vi "Backpressure - level-aware.vi"(8 "error in (no error)":errorcluster) -> (0 "error out":errorcluster)   [LabVIEW 2026, in "Tests.lvlib"]
doc: "Unit test (Caraya): verifies ApplyBackPressure's LevelAware policy, including the fast-path and scan oracle.\nOn a full bounded queue, asserts the victim is the oldest least-severe non-protected Statement (protected = level at or more severe than ERROR; floor = TRACE), that the incoming loses severity ties (strict worstSev > incoming), and that worstSeverityOut is recomputed over the survivors on the scan branch and passed through on the fast path.\nTests.lvlib, friend of Lumberjack.lvlib; unit tier.\n\nImplements LMBR-T-049 -> SRS-057. Assert-level IDs: Test-ID-Assert-Checklist.md."
uses:
  Tests.lvlib
  src/TypeDefs/Statement.ctl
  src/TypeDefs/Severity.ctl
  src/TypeDefs/DropPolicy.ctl
  <vilib>/addons/_JKI Toolkits/Caraya/classes/Assert/Assert Equal Value_Variant.vi
  <vilib>/addons/_JKI Toolkits/Caraya/classes/Test/Test.lvclass
  src/Lumberjack.lvlib
  <vilib>/addons/_JKI Toolkits/Caraya/classes/Assert/Assert.lvclass
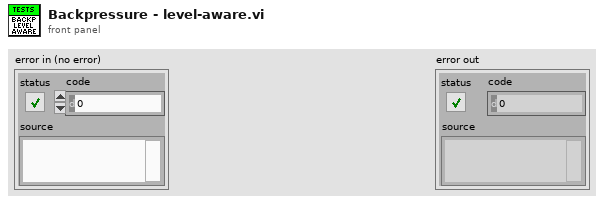
[diagram p1: front panel]
types:
  T1 = typedef "Lumberjack.lvlib/Statement.ctl" = cluster{"timestamp":timestamp, "level":T2, "sourceTag":string, "originVI":string, "message":string}
  T2 = typedef "Lumberjack.lvlib/Severity.ctl" = enum16{"OFF", "FATAL", "ERROR", "WARN", "INFO", "DEBUG", "TRACE", "ALL"}
  T3 = typedef "Lumberjack.lvlib/DropPolicy.ctl" = enum16{"DropOldest", "DropNewest", "LevelAware"}
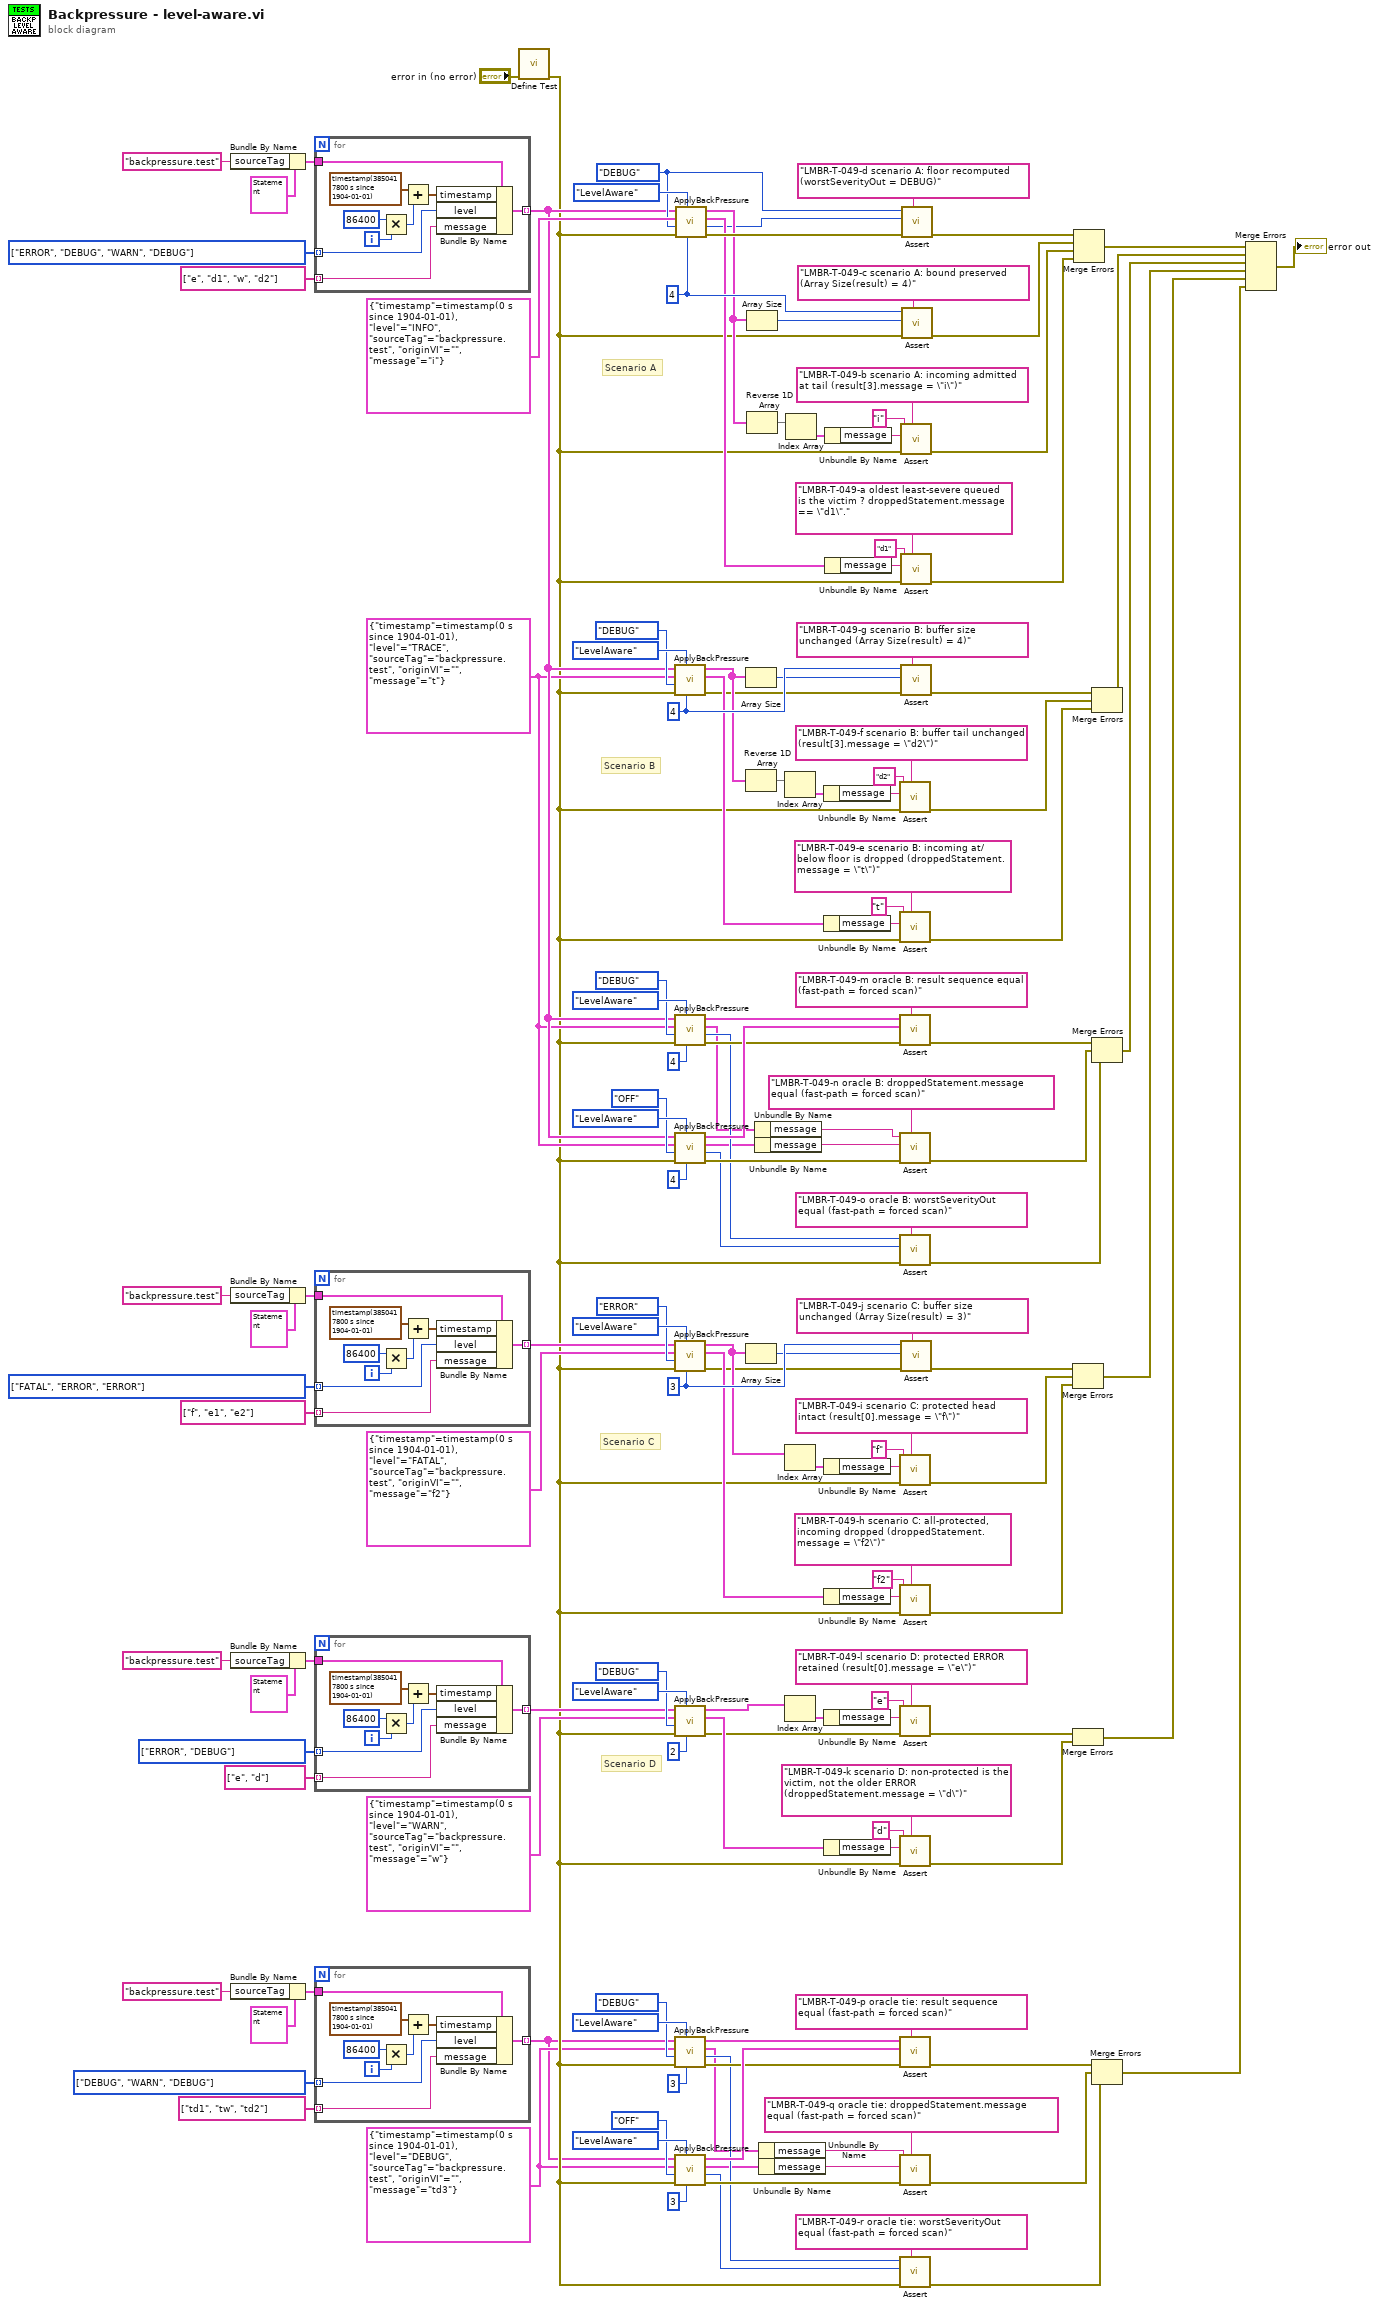
[diagram p0: block diagram]
diagram:
  w2 = T1 {"timestamp"=timestamp(0 s since 1904-01-01), "level"=enum."DEBUG", "sourceTag"="backpressure.test", "originVI"="", "message"="td3"} ("incoming")
  w12 = T2[] [enum."DEBUG", enum."WARN", enum."DEBUG"] items=["OFF", "FATAL", "ERROR", "WARN", "INFO", "DEBUG", "TRACE", "ALL"]
  w76 = T2[] [enum."ERROR", enum."DEBUG"] items=["OFF", "FATAL", "ERROR", "WARN", "INFO", "DEBUG", "TRACE", "ALL"]
  w98 = 3 ("queueBound")
  w101 = T2[] [enum."FATAL", enum."ERROR", enum."ERROR"] items=["OFF", "FATAL", "ERROR", "WARN", "INFO", "DEBUG", "TRACE", "ALL"]
  w51 = T1 {"timestamp"=timestamp(0 s since 1904-01-01), "level"=enum."TRACE", "sourceTag"="backpressure.test", "originVI"="", "message"="t"} ("incoming")
  w125 = 4 ("queueBound")
  w130 = T2[] [enum."ERROR", enum."DEBUG", enum."WARN", enum."DEBUG"] items=["OFF", "FATAL", "ERROR", "WARN", "INFO", "DEBUG", "TRACE", "ALL"]
  w129 = Severity."DEBUG" ("worstSeverityIn")
  w148 = 4 ("queueBound")
  # "Scenario D"
  # "Scenario C"
  # "Scenario B"
  # "Scenario A"
  n1 = Bundle By Name(cluster=T1 {"timestamp"=timestamp(0 s since 1904-01-01), "level"=enum."INFO", "sourceTag"="", "originVI"="", "message"=""} ("Statement"), "sourceTag"="backpressure.test") -> (w153:T1)
  n2 = Bundle By Name(cluster=T1 {"timestamp"=timestamp(0 s since 1904-01-01), "level"=enum."INFO", "sourceTag"="", "originVI"="", "message"=""} ("Statement"), "sourceTag"="backpressure.test") -> (w103:T1)
  n3 = Bundle By Name(cluster=T1 {"timestamp"=timestamp(0 s since 1904-01-01), "level"=enum."INFO", "sourceTag"="", "originVI"="", "message"=""} ("Statement"), "sourceTag"="backpressure.test") -> (w78:T1)
  n4 = Bundle By Name(cluster=T1 {"timestamp"=timestamp(0 s since 1904-01-01), "level"=enum."INFO", "sourceTag"="", "originVI"="", "message"=""} ("Statement"), "sourceTag"="backpressure.test") -> (w14:T1)
  n5 = for {
    tunnel: w153 -> [w162]
    tunnel: string[] ["e", "d1", "w", "d2"] -> [w159] mode=indexing
    tunnel: [w158] -> w52 mode=indexing
    tunnel: w130 -> [w157] mode=indexing
    i -> [w160]
    n6 = Multiply(x=86400, y=w160) -> (x*y=w164:i32)
    n7 = Add(x=timestamp(3850417800 s since 1904-01-01), y=w164) -> (x+y=w161:timestamp)
    n8 = Bundle By Name(cluster=w162, "timestamp"=w161, "level"=w157, "message"=w159) -> (w158:T1)
  }
  n9 = for {
    tunnel: w103 -> [w171]
    tunnel: string[] ["f", "e1", "e2"] -> [w168] mode=indexing
    tunnel: [w167] -> w84 mode=indexing
    tunnel: w101 -> [w166] mode=indexing
    i -> [w169]
    n10 = Multiply(x=86400, y=w169) -> (x*y=w173:i32)
    n11 = Add(x=timestamp(3850417800 s since 1904-01-01), y=w173) -> (x+y=w170:timestamp)
    n12 = Bundle By Name(cluster=w171, "timestamp"=w170, "level"=w166, "message"=w168) -> (w167:T1)
  }
  n13 = for {
    tunnel: w78 -> [w180]
    tunnel: string[] ["e", "d"] -> [w177] mode=indexing
    tunnel: [w176] -> w62 mode=indexing
    tunnel: w76 -> [w175] mode=indexing
    i -> [w178]
    n14 = Multiply(x=86400, y=w178) -> (x*y=w182:i32)
    n15 = Add(x=timestamp(3850417800 s since 1904-01-01), y=w182) -> (x+y=w179:timestamp)
    n16 = Bundle By Name(cluster=w180, "timestamp"=w179, "level"=w175, "message"=w177) -> (w176:T1)
  }
  n17 = for {
    tunnel: w14 -> [w189]
    tunnel: string[] ["td1", "tw", "td2"] -> [w186] mode=indexing
    tunnel: [w185] -> w1 mode=indexing
    tunnel: w12 -> [w184] mode=indexing
    i -> [w187]
    n18 = Multiply(x=86400, y=w187) -> (x*y=w191:i32)
    n19 = Add(x=timestamp(3850417800 s since 1904-01-01), y=w191) -> (x+y=w188:timestamp)
    n20 = Bundle By Name(cluster=w189, "timestamp"=w188, "level"=w184, "message"=w186) -> (w185:T1)
  }
  n21 = call <vilib>:"Define Test.vi"("error in (no error)"="error in (no error)") -> ("error out"=w11:errorcluster)  [unwired: 9 in, 1 out]
  n22 = call "ApplyBackPressure.vi"("queueBound"=w125, "DropPolicy"=DropPolicy."LevelAware", "error in (no error)"=w11, "worstSeverityIn"=Severity."DEBUG", "incoming"=w51, "pending"=w52) -> ("error out"=w106:errorcluster, "droppedStatement"=w121:T1, "result"=w114:T1[])  [unwired: 1 in, 2 out]
  n23 = call "ApplyBackPressure.vi"("queueBound"=4, "DropPolicy"=DropPolicy."LevelAware", "error in (no error)"=w11, "worstSeverityIn"=Severity."DEBUG", "incoming"=w51, "pending"=w52) -> ("error out"=w47:errorcluster, "worstSeverityOut"=w43:T2, "droppedStatement"=w10:T1, "result"=w49:T1[])  [unwired: 1 in, 1 out]
  n24 = call "ApplyBackPressure.vi"("queueBound"=4, "DropPolicy"=DropPolicy."LevelAware", "error in (no error)"=w11, "worstSeverityIn"=Severity."OFF", "incoming"=w51, "pending"=w52) -> ("error out"=w45:errorcluster, "worstSeverityOut"=w42:T2, "droppedStatement"=w9:T1, "result"=w48:T1[])  [unwired: 1 in, 1 out]
  n25 = call "ApplyBackPressure.vi"("queueBound"=w98, "DropPolicy"=DropPolicy."LevelAware", "error in (no error)"=w11, "worstSeverityIn"=Severity."ERROR", "incoming"=T1 {"timestamp"=timestamp(0 s since 1904-01-01), "level"=enum."FATAL", "sourceTag"="backpressure.test", "originVI"="", "message"="f2"}, "pending"=w84) -> ("error out"=w81:errorcluster, "droppedStatement"=w94:T1, "result"=w82:T1[])  [unwired: 1 in, 2 out]
  n26 = call "ApplyBackPressure.vi"("queueBound"=2, "DropPolicy"=DropPolicy."LevelAware", "error in (no error)"=w11, "worstSeverityIn"=Severity."DEBUG", "incoming"=T1 {"timestamp"=timestamp(0 s since 1904-01-01), "level"=enum."WARN", "sourceTag"="backpressure.test", "originVI"="", "message"="w"}, "pending"=w62) -> ("error out"=w59:errorcluster, "droppedStatement"=w71:T1, "result"=w60:T1[])  [unwired: 1 in, 2 out]
  n27 = call "ApplyBackPressure.vi"("queueBound"=3, "DropPolicy"=DropPolicy."LevelAware", "error in (no error)"=w11, "worstSeverityIn"=Severity."DEBUG", "incoming"=w2, "pending"=w1) -> ("error out"=w27:errorcluster, "worstSeverityOut"=w23:T2, "droppedStatement"=w4:T1, "result"=w29:T1[])  [unwired: 1 in, 1 out]
  n28 = call "ApplyBackPressure.vi"("queueBound"=3, "DropPolicy"=DropPolicy."LevelAware", "error in (no error)"=w11, "worstSeverityIn"=Severity."OFF", "incoming"=w2, "pending"=w1) -> ("error out"=w25:errorcluster, "worstSeverityOut"=w22:T2, "droppedStatement"=w6:T1, "result"=w28:T1[])  [unwired: 1 in, 1 out]
  n29 = call "ApplyBackPressure.vi"("queueBound"=w148, "DropPolicy"=DropPolicy."LevelAware", "error in (no error)"=w11, "worstSeverityIn"=w129, "incoming"=T1 {"timestamp"=timestamp(0 s since 1904-01-01), "level"=enum."INFO", "sourceTag"="backpressure.test", "originVI"="", "message"="i"}, "pending"=w52) -> ("error out"=w150:errorcluster, "worstSeverityOut"=w128:T2, "droppedStatement"=w143:T1, "result"=w134:T1[])  [unwired: 1 in, 1 out]
  n30 = Array Size(array=w114) -> (size(s)=w124:i32)
  n31 = Reverse 1D Array(array=w114) -> (reversed array=w119:T1[])
  n32 = Array Size(array=w82) -> (size(s)=w97:i32)
  n33 = Array Size(array=w134) -> (size(s)=w147:i32)
  n34 = Reverse 1D Array(array=w134) -> (reversed array=w139:T1[])
  n35 = Unbundle By Name(w10) -> ("message"=w7:string)
  n36 = Unbundle By Name(w9) -> ("message"=w8:string)
  n37 = Unbundle By Name(w4) -> ("message"=w3:string)
  n38 = Unbundle By Name(w6) -> ("message"=w5:string)
  n39 = Index Array(array=w119) -> (element=w115:T1)  [unwired: 1 in]
  n40 = Index Array(array=w82) -> (element=w88:T1)  [unwired: 1 in]
  n41 = Index Array(array=w60) -> (element=w66:T1)  [unwired: 1 in]
  n42 = Index Array(array=w139) -> (element=w135:T1)  [unwired: 1 in]
  n43 = Unbundle By Name(w115) -> ("message"=w116:string)
  n44 = Unbundle By Name(w121) -> ("message"=w120:string)
  n45 = Unbundle By Name(w88) -> ("message"=w89:string)
  n46 = Unbundle By Name(w94) -> ("message"=w93:string)
  n47 = Unbundle By Name(w66) -> ("message"=w67:string)
  n48 = Unbundle By Name(w71) -> ("message"=w70:string)
  n49 = Unbundle By Name(w135) -> ("message"=w136:string)
  n50 = Unbundle By Name(w143) -> ("message"=w142:string)
  n51 = call-poly <vilib>:"Assert.vi"("Label"="LMBR-T-049-f scenario B: buffer tail unchanged (result[3].message = \"d2\")" ("sourceTag"), "error in (no error)"=w11, "Actual"=w116, "Expected"="d2") -> ("error out"=w111:errorcluster)  [unwired: 6 in, 1 out]
  n52 = call-poly <vilib>:"Assert.vi"("Label"="LMBR-T-049-e scenario B: incoming at/below floor is dropped (droppedStatement.message = \"t\")" ("sourceTag"), "error in (no error)"=w11, "Actual"=w120, "Expected"="t") -> ("error out"=w110:errorcluster)  [unwired: 6 in, 1 out]
  n53 = call-poly <vilib>:"Assert.vi"("Label"="LMBR-T-049-m oracle B: result sequence equal (fast-path = forced scan)" ("sourceTag"), "error in (no error)"=w47, "Actual"=w48, "Expected"=w49) -> ("error out"=w41:errorcluster)  [unwired: 6 in, 1 out]
  n54 = call-poly <vilib>:"Assert.vi"("Label"="LMBR-T-049-n oracle B: droppedStatement.message equal (fast-path = forced scan)" ("sourceTag"), "error in (no error)"=w45, "Actual"=w8, "Expected"=w7) -> ("error out"=w40:errorcluster)  [unwired: 6 in, 1 out]
  n55 = call-poly <vilib>:"Assert.vi"("Label"="LMBR-T-049-o oracle B: worstSeverityOut equal (fast-path = forced scan)" ("sourceTag"), "error in (no error)"=w11, "Actual"=w42, "Expected"=w43) -> ("error out"=w39:errorcluster)  [unwired: 6 in, 1 out]
  n56 = call-poly <vilib>:"Assert.vi"("Label"="LMBR-T-049-i scenario C: protected head intact (result[0].message = \"f\")" ("sourceTag"), "error in (no error)"=w11, "Actual"=w89, "Expected"="f") -> ("error out"=w87:errorcluster)  [unwired: 6 in, 1 out]
  n57 = call-poly <vilib>:"Assert.vi"("Label"="LMBR-T-049-h scenario C: all-protected, incoming dropped (droppedStatement.message = \"f2\")" ("sourceTag"), "error in (no error)"=w11, "Actual"=w93, "Expected"="f2") -> ("error out"=w86:errorcluster)  [unwired: 6 in, 1 out]
  n58 = call-poly <vilib>:"Assert.vi"("Label"="LMBR-T-049-l scenario D: protected ERROR retained (result[0].message = \"e\")" ("sourceTag"), "error in (no error)"=w59, "Actual"=w67, "Expected"="e") -> ("error out"=w65:errorcluster)  [unwired: 6 in, 1 out]
  n59 = call-poly <vilib>:"Assert.vi"("Label"="LMBR-T-049-k scenario D: non-protected is the victim, not the older ERROR (droppedStatement.message = \"d\")" ("sourceTag"), "error in (no error)"=w11, "Actual"=w70, "Expected"="d") -> ("error out"=w64:errorcluster)  [unwired: 6 in, 1 out]
  n60 = call-poly <vilib>:"Assert.vi"("Label"="LMBR-T-049-p oracle tie: result sequence equal (fast-path = forced scan)" ("sourceTag"), "error in (no error)"=w27, "Actual"=w28, "Expected"=w29) -> ("error out"=w21:errorcluster)  [unwired: 6 in, 1 out]
  n61 = call-poly <vilib>:"Assert.vi"("Label"="LMBR-T-049-q oracle tie: droppedStatement.message equal (fast-path = forced scan)" ("sourceTag"), "error in (no error)"=w25, "Actual"=w5, "Expected"=w3) -> ("error out"=w20:errorcluster)  [unwired: 6 in, 1 out]
  n62 = call-poly <vilib>:"Assert.vi"("Label"="LMBR-T-049-r oracle tie: worstSeverityOut equal (fast-path = forced scan)" ("sourceTag"), "error in (no error)"=w11, "Actual"=w22, "Expected"=w23) -> ("error out"=w19:errorcluster)  [unwired: 6 in, 1 out]
  n63 = call-poly <vilib>:"Assert.vi"("Label"="LMBR-T-049-b scenario A: incoming admitted at tail (result[3].message = \"i\")" ("sourceTag"), "error in (no error)"=w11, "Actual"=w136, "Expected"="i") -> ("error out"=w133:errorcluster)  [unwired: 6 in, 1 out]
  n64 = call-poly <vilib>:"Assert.vi"("Label"="LMBR-T-049-a oldest least-severe queued is the victim ? droppedStatement.message == \"d1\"." ("sourceTag"), "error in (no error)"=w11, "Actual"=w142, "Expected"="d1") -> ("error out"=w132:errorcluster)  [unwired: 6 in, 1 out]
  n65 = call-poly <vilib>:"Assert.vi"("Label"="LMBR-T-049-g scenario B: buffer size unchanged (Array Size(result) = 4)" ("sourceTag"), "error in (no error)"=w106, "Actual"=w124, "Expected"=w125) -> ("error out"=w112:errorcluster)  [unwired: 6 in, 1 out]
  n66 = call-poly <vilib>:"Assert.vi"("Label"="LMBR-T-049-j scenario C: buffer size unchanged (Array Size(result) = 3)" ("sourceTag"), "error in (no error)"=w81, "Actual"=w97, "Expected"=w98) -> ("error out"=w92:errorcluster)  [unwired: 6 in, 1 out]
  n67 = call-poly <vilib>:"Assert.vi"("Label"="LMBR-T-049-d scenario A: floor recomputed (worstSeverityOut = DEBUG)" ("sourceTag"), "error in (no error)"=w150, "Actual"=w128, "Expected"=w129) -> ("error out"=w141:errorcluster)  [unwired: 6 in, 1 out]
  n68 = call-poly <vilib>:"Assert.vi"("Label"="LMBR-T-049-c scenario A: bound preserved (Array Size(result) = 4)" ("sourceTag"), "error in (no error)"=w11, "Actual"=w147, "Expected"=w148) -> ("error out"=w140:errorcluster)  [unwired: 6 in, 1 out]
  n69 = Merge Errors(w92, w87, w86) -> (w37:errorcluster)
  n70 = Merge Errors(w65, w64) -> (w18:errorcluster)
  n71 = Merge Errors(w141, w140, w133, w132) -> (w109:errorcluster)
  n72 = Merge Errors(w112, w111, w110) -> (w107:errorcluster)
  n73 = Merge Errors(w41, w40, w39) -> (w38:errorcluster)
  n74 = Merge Errors(w21, w20, w19) -> (w17:errorcluster)
  n75 = Merge Errors(w109, w107, w38, w37, w18, w17) -> (→"error out":errorcluster)
